vi "Get Error.vi"(7 "timeout (1s)":dbl=1.0 min=0.0, 8 "error in (no error)":errorcluster, 11 "SDO object in":refnum<k20>) -> (0 "error out":errorcluster, 1 "completion code":u32 format="%.0x", 2 "Error code":u16, 3 "SDO object out":refnum<k20>, 5 "Error register":u8)   [LabVIEW 2016]
uses:
  <vilib>/CANopenLib/CANOPEN.llb/CANopen SDO Read [U16].vi
  <vilib>/CANopenLib/CANOPEN.llb/CANopen SDO Read [U8].vi
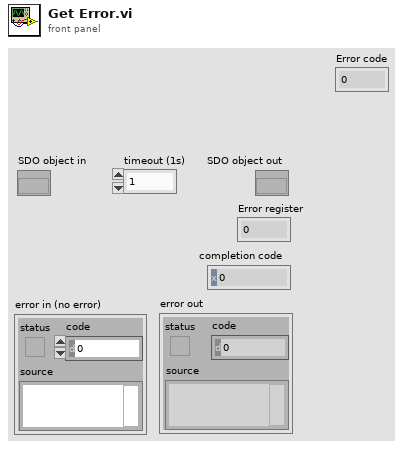
[diagram p1: front panel]
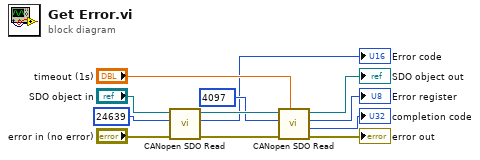
[diagram p0: block diagram]
diagram:
  n1 = call-poly <vilib>:"CANopen SDO Read.vi"("error in (no error)"="error in (no error)", "object index"=u16 24639, "SDO object in"="SDO object in") -> ("error out"=w6:errorcluster, "U16 data"=→"Error code":u16, "SDO object out"=w5:refnum<k20>)  [unwired: 5 in, 1 out]
  n2 = call-poly <vilib>:"CANopen SDO Read.vi"("timeout (1s)"="timeout (1s)", "error in (no error)"=w6, "object index"=u16 4097, "SDO object in"=w5) -> ("error out"=→"error out":errorcluster, "completion code"=→"completion code":u32, "U8 data"=→"Error register":u8, "SDO object out"=→"SDO object out":refnum<k20>)  [unwired: 4 in]
